vi "AlazarBoardsInSystemByHandle.vi"(0 "Handle":u64, 1 "error in (no error)":errorcluster) -> (2 "Handle":u64, 3 "Board Count":u32, 5 "error out":errorcluster)   [LabVIEW 2018]
doc: "Return the number of digitizer boards in a board system specified by the handle of its master board."
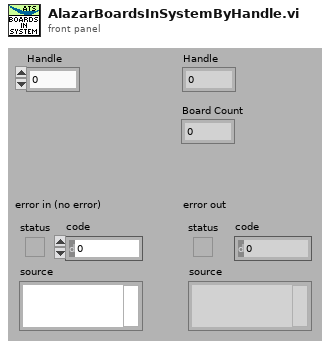
[diagram p1: front panel]
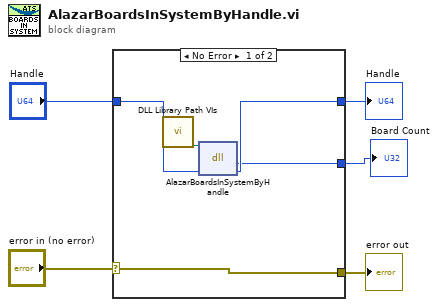
[diagram p0: block diagram]
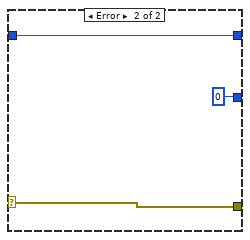
[diagram p2: hidden frame]
diagram:
  n1 = case shown="No Error" "error in (no error)" {
    selector: "error in (no error)" -> [w8 w13]
    tunnel: [w8 w13] -> w4
    tunnel: "Handle" -> [w10 w12]
    tunnel: [w9 w12] -> w2
    tunnel: [w7 u32 0] -> w1
    frame No Error {
      n2 = call "DLL Library Path VIs.vi"() -> ("Alazar"=w6:path)  [unwired: 9 in, 2 out]
      n3 = dll-call lib="C:/Project/SerialSectOCT - FFT GPU/SerialSectOCT/Labview Software/DLL/ATSApi.dll" fn="AlazarBoardsInSystemByHandle"(path in=w6, "handle"=w10) -> ("return type"=w7:u32, "handle"=w9:u64)  [unwired: 2 in, 2 out]
    }
    frame Error {
    }
  }
  "Handle" <- w2
  "error out" <- w4
  "Board Count" <- w1
